vi "Parse_tags_to_DPP.vi"(11 "XML":string) -> (2 "DPP Configuration":T1)   [LabVIEW 2015]
uses:
  ConfigurationDPP.ctl
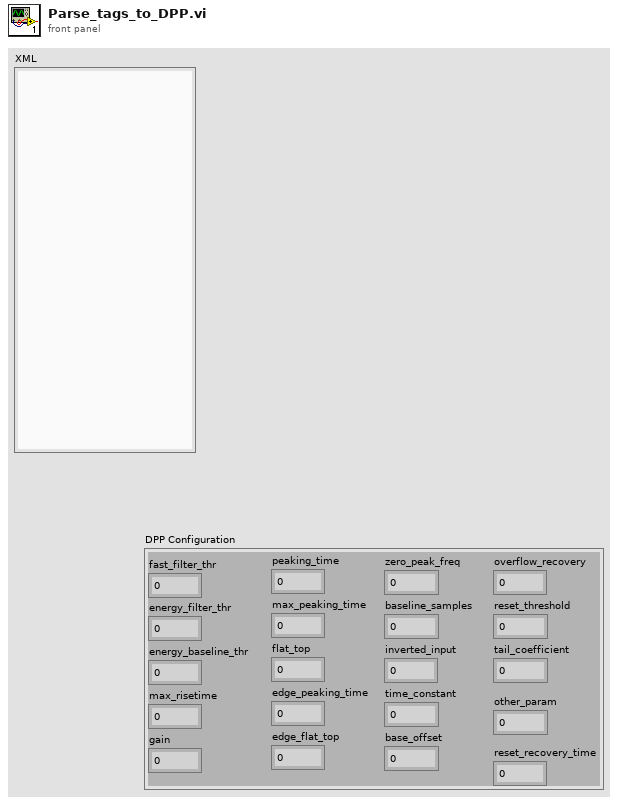
[diagram p1: front panel]
types:
  T1 = typedef "ConfigurationDPP.ctl" = cluster{"reset_recovery_time":u32, "edge_peaking_time":u32, "flat_top":u32, "peaking_time":u32, "gain":dbl, "max_risetime":dbl, "fast_filter_thr":u32, "zero_peak_freq":dbl, "inverted_input":u8, "base_offset":u32, "reset_threshold":u32, "overflow_recovery":u32, "tail_coefficient":dbl, "energy_filter_thr":u32, "energy_baseline_thr":u32, "max_peaking_time":u32, "edge_flat_top":u32, "time_constant":dbl, "baseline_samples":u32, "other_param":u32}
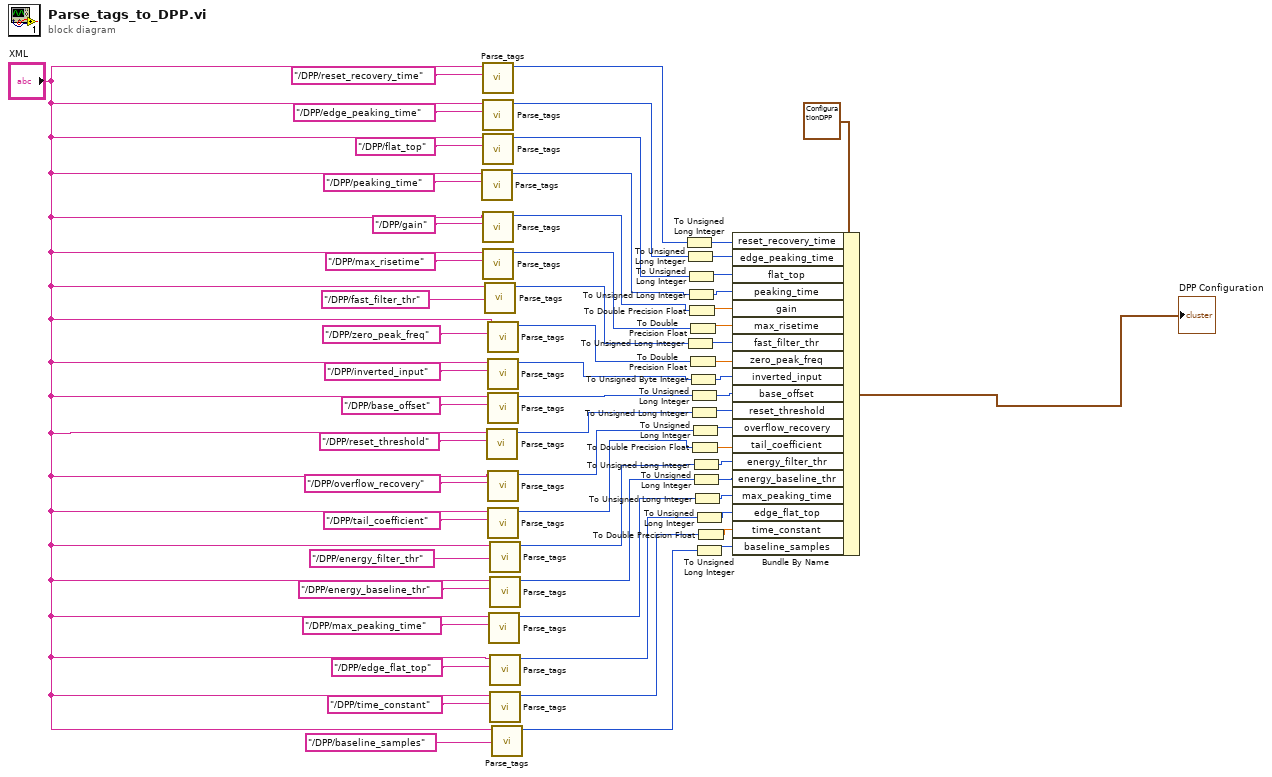
[diagram p0: block diagram]
diagram:
  n1 = call "Parse_tags.vi"("XPath expression"="/DPP/peaking_time", "XML"="XML") -> ("String"=w43:i32)  [unwired: 9 in]
  n2 = call "Parse_tags.vi"("XPath expression"="/DPP/reset_recovery_time", "XML"="XML") -> ("String"=w54:i32)  [unwired: 9 in]
  n3 = call "Parse_tags.vi"("XPath expression"="/DPP/edge_peaking_time", "XML"="XML") -> ("String"=w51:i32)  [unwired: 9 in]
  n4 = call "Parse_tags.vi"("XPath expression"="/DPP/flat_top", "XML"="XML") -> ("String"=w46:i32)  [unwired: 9 in]
  n5 = call "Parse_tags.vi"("XPath expression"="/DPP/gain", "XML"="XML") -> ("String"=w41:i32)  [unwired: 9 in]
  n6 = call "Parse_tags.vi"("XPath expression"="/DPP/max_risetime", "XML"="XML") -> ("String"=w38:i32)  [unwired: 9 in]
  n7 = call "Parse_tags.vi"("XPath expression"="/DPP/fast_filter_thr", "XML"="XML") -> ("String"=w59:i32)  [unwired: 9 in]
  n8 = call "Parse_tags.vi"("XPath expression"="/DPP/reset_threshold", "XML"="XML") -> ("String"=w26:i32)  [unwired: 9 in]
  n9 = call "Parse_tags.vi"("XPath expression"="/DPP/zero_peak_freq", "XML"="XML") -> ("String"=w30:i32)  [unwired: 9 in]
  n10 = call "Parse_tags.vi"("XPath expression"="/DPP/inverted_input", "XML"="XML") -> ("String"=w1:i32)  [unwired: 9 in]
  n11 = call "Parse_tags.vi"("XPath expression"="/DPP/base_offset", "XML"="XML") -> ("String"=w28:i32)  [unwired: 9 in]
  n12 = call "Parse_tags.vi"("XPath expression"="/DPP/overflow_recovery", "XML"="XML") -> ("String"=w23:i32)  [unwired: 9 in]
  n13 = call "Parse_tags.vi"("XPath expression"="/DPP/tail_coefficient", "XML"="XML") -> ("String"=w22:i32)  [unwired: 9 in]
  n14 = call "Parse_tags.vi"("XPath expression"="/DPP/max_peaking_time", "XML"="XML") -> ("String"=w9:i32)  [unwired: 9 in]
  n15 = call "Parse_tags.vi"("XPath expression"="/DPP/energy_filter_thr", "XML"="XML") -> ("String"=w19:i32)  [unwired: 9 in]
  n16 = call "Parse_tags.vi"("XPath expression"="/DPP/energy_baseline_thr", "XML"="XML") -> ("String"=w12:i32)  [unwired: 9 in]
  n17 = call "Parse_tags.vi"("XPath expression"="/DPP/edge_flat_top", "XML"="XML") -> ("String"=w7:i32)  [unwired: 9 in]
  n18 = call "Parse_tags.vi"("XPath expression"="/DPP/time_constant", "XML"="XML") -> ("String"=w5:i32)  [unwired: 9 in]
  n19 = call "Parse_tags.vi"("XPath expression"="/DPP/baseline_samples", "XML"="XML") -> ("String"=w3:i32)  [unwired: 9 in]
  n20 = To Unsigned Long Integer(number=w54) -> (unsigned 32bit integer=w53:u32)
  n21 = To Unsigned Long Integer(number=w51) -> (unsigned 32bit integer=w50:u32)
  n22 = To Unsigned Long Integer(number=w59) -> (unsigned 32bit integer=w60:u32)
  n23 = To Unsigned Long Integer(number=w46) -> (unsigned 32bit integer=w47:u32)
  n24 = To Unsigned Long Integer(number=w43) -> (unsigned 32bit integer=w44:u32)
  n25 = To Double Precision Float(number=w41) -> (double precision float=w42:dbl)
  n26 = To Double Precision Float(number=w38) -> (double precision float=w39:dbl)
  n27 = To Double Precision Float(number=w30) -> (double precision float=w29:dbl)
  n28 = To Unsigned Byte Integer(number=w1) -> (unsigned 8bit integer=w2:u8)
  n29 = To Unsigned Long Integer(number=w28) -> (unsigned 32bit integer=w27:u32)
  n30 = To Unsigned Long Integer(number=w26) -> (unsigned 32bit integer=w25:u32)
  n31 = To Unsigned Long Integer(number=w23) -> (unsigned 32bit integer=w24:u32)
  n32 = To Double Precision Float(number=w22) -> (double precision float=w21:dbl)
  n33 = To Unsigned Long Integer(number=w19) -> (unsigned 32bit integer=w20:u32)
  n34 = To Unsigned Long Integer(number=w12) -> (unsigned 32bit integer=w11:u32)
  n35 = To Unsigned Long Integer(number=w9) -> (unsigned 32bit integer=w10:u32)
  n36 = To Unsigned Long Integer(number=w7) -> (unsigned 32bit integer=w8:u32)
  n37 = To Unsigned Long Integer(number=w3) -> (unsigned 32bit integer=w4:u32)
  n38 = To Double Precision Float(number=w5) -> (double precision float=w6:dbl)
  n39 = Bundle By Name(cluster=T1 {"reset_recovery_time"=300, "edge_peaking_time"=5, "flat_top"=5, "peaking_time"=25, "gain"=1.0, "max_risetime"=35.0, "fast_filter_thr"=100, "zero_peak_freq"=5.0, "inverted_input"=0, "base_offset"=0, "reset_threshold"=1000, "overflow_recovery"=0, "tail_coefficient"=0.0, "energy_filter_thr"=25, "energy_baseline_thr"=25, "max_peaking_time"=0, "edge_flat_top"=1, "time_constant"=0.0, "baseline_samples"=64, "other_param"=0} ("DPP Configuration"), "reset_recovery_time"=w53, "edge_peaking_time"=w50, "flat_top"=w47, "peaking_time"=w44, "gain"=w42, "max_risetime"=w39, "fast_filter_thr"=w60, "zero_peak_freq"=w29, "inverted_input"=w2, "base_offset"=w27, "reset_threshold"=w25, "overflow_recovery"=w24, "tail_coefficient"=w21, "energy_filter_thr"=w20, "energy_baseline_thr"=w11, "max_peaking_time"=w10, "edge_flat_top"=w8, "time_constant"=w6, "baseline_samples"=w4) -> (→"DPP Configuration":T1)
